vi "ColorToRGB.vi"(5 "color":u32(colorbox)) -> (0 "transparent?":bool, 1 "blue":u8, 2 "green":u8, 3 "red":u8)   [LabVIEW 2015, in "NI_ReportGenerationCore.lvlib"]
doc: "Non-API VI."
uses:
  <vilib>/Utility/NIReport.llb/NI_ReportGenerationCore.lvlib
panel:
  out "Color-Cluster":T1
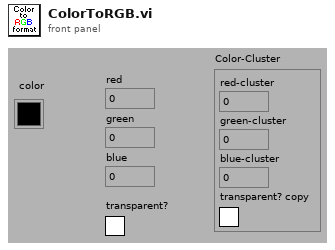
[diagram p1: front panel]
types:
  T1 = cluster{"red-cluster":u8, "green-cluster":u8, "blue-cluster":u8, "transparent? copy":bool}
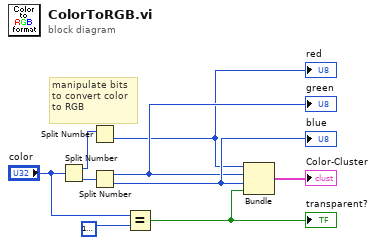
[diagram p0: block diagram]
diagram:
  # "manipulate bits\nto convert color\nto RGB"
  n1 = Split Number(x="color") -> (hi(x)=w3:u16, lo(x)=w2:u16)
  n2 = Split Number(x=w3) -> (lo(x)=w7:u8)  [unwired: 1 out]
  "red" <- w7
  n3 = Split Number(x=w2) -> (hi(x)=w8:u8, lo(x)=w9:u8)
  "blue" <- w9
  "green" <- w8
  n4 = Equal?(x="color", y=u32 16777216 ("color")) -> (x = y?=w4:bool)
  "transparent?" <- w4
  n5 = Bundle(w7, w8, w9, w4) -> (→"Color-Cluster":cluster{u8, u8, u8, bool})  [unwired: 1 in]
